vi "Auto_Routine_LeftTwoPieceTRAJ.vi"   [LabVIEW 2023]
uses:
  Arm2/ArmGetSetpointEnum.ctl
  Trajectory/TrajectoryGlobals.vi
  <vilib>/Rock Robotics/WPI/ThirdParty/JAS_Junk/TrajLib/Trajectory_Library.lvlib
types:
  T1 = typedef "ArmGetSetpointEnum.ctl" = enum16{"ArmFloorPickup", "ArmAmpDeposit", "ArmSpeakerShoot", "ArmStartPosition", "ArmRestPosition", "ArmSourceIntake", "ArmAwayShoot"}
  T2 = typedef "Trajectory_Library.lvlib/TRAJECTORY.ctl" = cluster{"TotalTImeSecs":dbl, "States":T3[]}
  T3 = typedef "Trajectory_Library.lvlib/TRAJ_STATE.ctl" = cluster{"TimeSeconds":dbl, "Velocity":dbl, "Acceleration":dbl, "POSE":T4, "Curvature":dbl}
  T4 = typedef "Trajectory_Library.lvlib/POSE2D.ctl" = cluster{"TRANSLATION":T5, "ROTATION":T6}
  T5 = typedef "Trajectory_Library.lvlib/TRANSLATION2D.ctl" = cluster{"X":dbl, "Y":dbl}
  T6 = typedef "Trajectory_Library.lvlib/ROTATION2D.ctl" = cluster{"VALUE":dbl, "COS":dbl, "SIN":dbl}
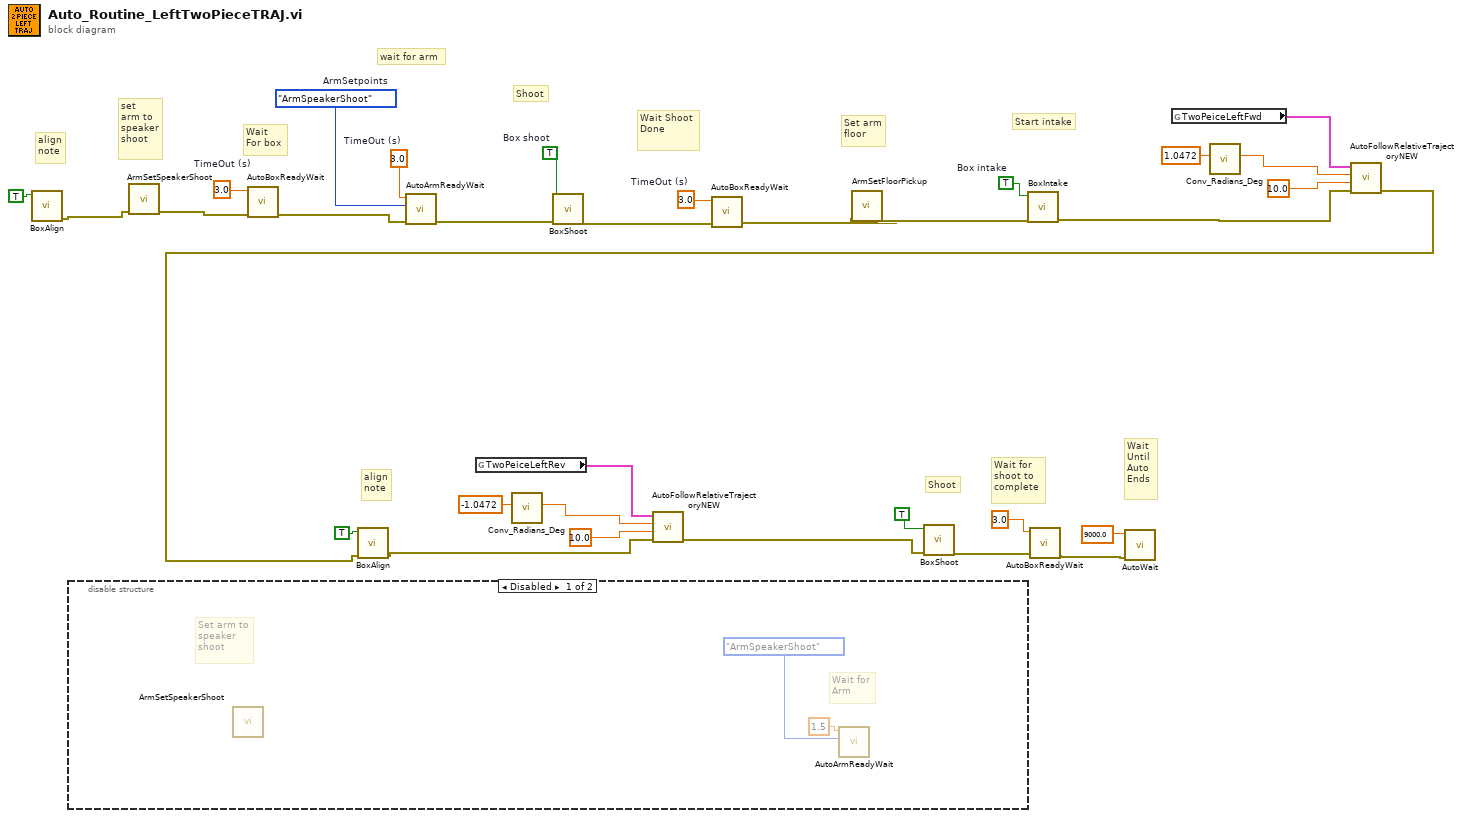
[diagram p0: block diagram]
diagram:
  w22 = 3.0  # TimeOut (s)
  w32 = TRUE  # Box intake
  w31 = TRUE  # Box shoot
  w30 = ArmGetSetpointEnum."ArmSpeakerShoot"  # ArmSetpoints
  w29 = 3.0  # TimeOut (s)
  w25 = 3.0  # TimeOut (s)
  # "align\nnote"
  # "Wait\nUntil\nAuto \nEnds"
  # "Wait for\nshoot to\ncomplete"
  # "Shoot"
  # "Start intake"
  # "Set arm\nfloor"
  # "Wait Shoot\nDone"
  # "Shoot"
  # "Wait\nFor box"
  # "set \narm to\nspeaker\nshoot"
  # "align\nnote"
  # "wait for arm"
  n1 = call "BoxAlign.vi"("box align"=TRUE) -> ("error out"=w23:errorcluster)  [unwired: 10 in]
  n2 = disable-structure shown="Disabled" {
    frame Disabled {
      # "Wait for\nArm"
      # "Set arm to\nspeaker \nshoot"
      n3 = call "ArmSetSpeakerShoot.vi"() -> ()  [unwired: 11 in, 1 out]
      n4 = call "AutoArmReadyWait.vi"("ArmSetpoints"=ArmGetSetpointEnum."ArmSpeakerShoot", "TimeOut (s)"=1.5) -> ("error out"=w34:errorcluster, "error in (no error)"=w33:errorcluster)  [unwired: 8 in]
    }
    frame Enabled {
    }
  }
  n5 = call "ArmSetSpeakerShoot.vi"("error in (no error)"=w23) -> ("error out"=w21:errorcluster)  [unwired: 10 in]
  n6 = call "AutoBoxReadyWait.vi"("error in (no error)"=w21, "TimeOut (s)"=w22) -> ("error out"=w20:errorcluster)  [unwired: 9 in]
  n7 = call "AutoArmReadyWait.vi"("error in (no error)"=w20, "ArmSetpoints"=w30, "TimeOut (s)"=w29) -> ("error out"=w26:errorcluster)  [unwired: 8 in]
  n8 = global read "TrajectoryGlobals.vi" "TwoPeiceLeftRev"() -> (w9:T2)
  n9 = call <vilib>:"Conv_Radians_Deg.vi"("Radians"=-1.0472) -> ("Degrees"=w7:dbl)  [unwired: 10 in]
  n10 = call "BoxShoot.vi"("error in (no error)"=w26, "Box shoot"=w31) -> ("error out"=w27:errorcluster)  [unwired: 9 in]
  n11 = call "AutoBoxReadyWait.vi"("error in (no error)"=w27, "TimeOut (s)"=w25) -> ("error out"=w19:errorcluster)  [unwired: 9 in]
  n12 = call "ArmSetFloorPickup.vi"("error in (no error)"=w19) -> ("error out"=w28:errorcluster)  [unwired: 10 in]
  n13 = call "BoxIntake.vi"("error in (no error)"=w28, "Box intake"=w32) -> ("error out"=w18:errorcluster)  [unwired: 9 in]
  n14 = global read "TrajectoryGlobals.vi" "TwoPeiceLeftFwd"() -> (w17:T2)
  n15 = call <vilib>:"Conv_Radians_Deg.vi"("Radians"=1.0472) -> ("Degrees"=w15:dbl)  [unwired: 10 in]
  n16 = call "AutoFollowRelativeTrajectoryNEW.vi"("error in (no error)"=w18, "TimeOut (s)"=10.0, "End Orientation"=w15, "Trajectory"=w17) -> ("error out"=w2:errorcluster)  [unwired: 7 in]
  n17 = call "BoxAlign.vi"("error in (no error)"=w2, "box align"=TRUE) -> ("error out"=w3:errorcluster)  [unwired: 9 in]
  n18 = call "AutoFollowRelativeTrajectoryNEW.vi"("error in (no error)"=w3, "TimeOut (s)"=10.0, "End Orientation"=w7, "Trajectory"=w9) -> ("error out"=w1:errorcluster)  [unwired: 7 in]
  n19 = call "BoxShoot.vi"("error in (no error)"=w1, "Box shoot"=TRUE) -> ("error out"=w12:errorcluster)  [unwired: 9 in]
  n20 = call "AutoBoxReadyWait.vi"("error in (no error)"=w12, "TimeOut (s)"=3.0) -> ("error out"=w5:errorcluster)  [unwired: 9 in]
  n21 = call "AutoWait.vi"("error in (no error)"=w5, "TimeOut (s)"=9000.0) -> ()  [unwired: 9 in, 1 out]
